vi "CCDImageHL.vi"(0 "Type of Symmetry":u32(ring)=5 items=["Horizontal", "Vertical", "Central", "1st Diagonal", "2nd Diagonal", "No change"], 1 "Stop (F)":bool, 3 "Exposure::Mode":u32(ring)=2 items=["Auto"=1, "Manual"=2], 5 "Angle (degrees)":sgl(slide) scale=0.0..360.0, 9 "Image Logging Path":path=path "E:/ccd", 11 "Image Logging Prefix":string="Pupil", 12 "Log Image":bool, 14 "Exposure::Value":dbl=0.0625 min=0.0001220703125 max=0.5, 15 "error in":errorcluster) -> (4 "Transformed Image":T1(plugin-control) caption="Image", 6 "Image Number":u32=165, 8 "Frame Rate":dbl=12.609117361784675, 10 "Image Logging Path Out":path)   [LabVIEW 2016]
uses:
  <vilib>/vision/NI_Vision_Development_Module.lvlib
panel:
  out "error out":errorcluster
  out "RawImage":T1(plugin-control) caption="Image"
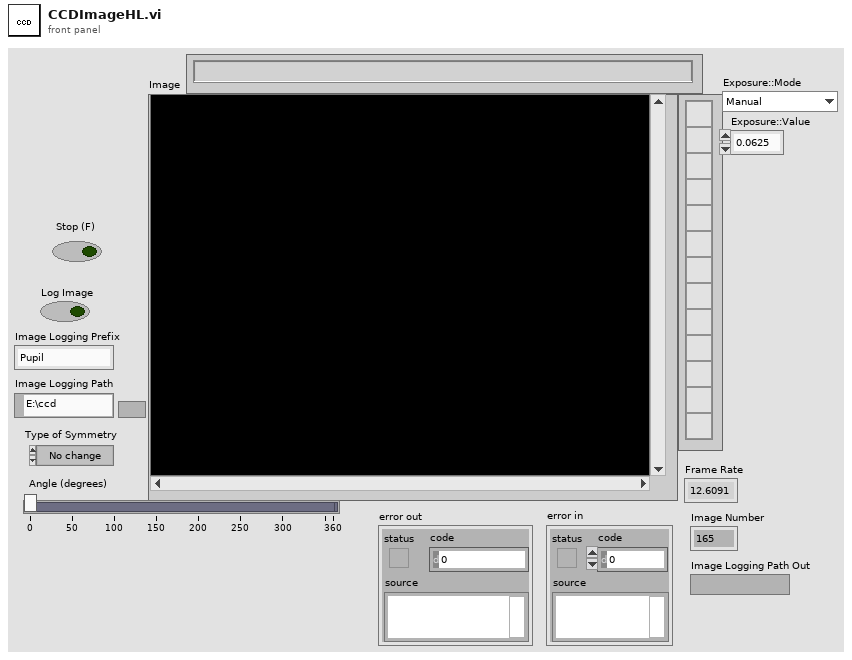
[diagram p1: front panel]
types:
  T1 = typedef "IMAQ Image.ctl" = refnum<image>
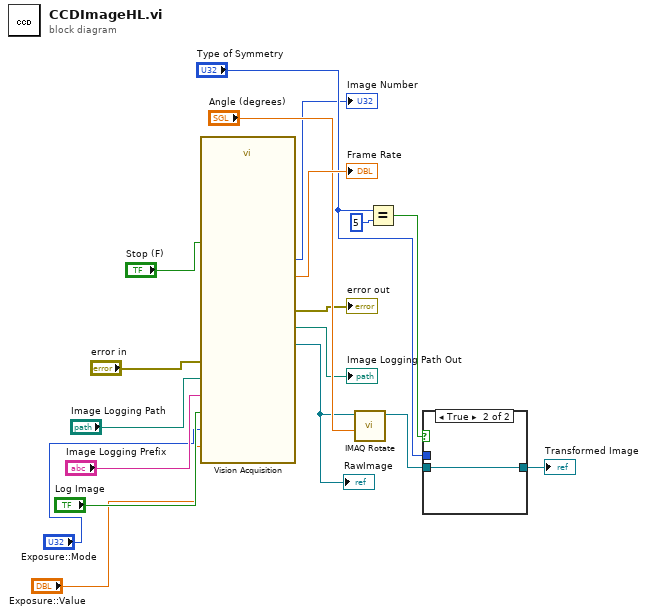
[diagram p0: block diagram]
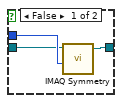
[diagram p2: hidden frame]
diagram:
  n1 = call "Vision Acquisition"("Log Image"="Log Image", "Image Logging Path"="Image Logging Path", "Image Logging Prefix"="Image Logging Prefix", "Exposure::Mode"="Exposure::Mode", "Exposure::Value"="Exposure::Value", "Stop (F)"="Stop (F)", "error in"="error in") -> ("Image Out"=w10:T1, "Image Number"=→"Image Number":u32, "Image Logging Path Out"=→"Image Logging Path Out":path, "Frame Rate"=→"Frame Rate":dbl, "error out"=→"error out":errorcluster)  [unwired: 15 in, 1 out]
  "RawImage" <- w10
  n2 = call "IMAQ Rotate"("Angle (degrees)"="Angle (degrees)", "Image Src"=w10) -> ("Image Dst Out"=w15:T1)  [unwired: 8 in, 1 out]
  n3 = Equal?(x="Type of Symmetry", y=u32 5) -> (x = y?=w11:bool)
  n4 = case shown="True" w11 {
    tunnel: "Type of Symmetry" -> [w21 _]
    tunnel: w15 -> [w20 w22]
    tunnel: [w19 w22] -> w14
    frame False {
      n5 = call "IMAQ Symmetry"("Type of Symmetry"=w21, "Image Src"=w20) -> ("Image Dst Out"=w19:T1)  [unwired: 3 in, 1 out]
    }
    frame True {
    }
  }
  "Transformed Image" <- w14
